vi "RXMux-DM.vi"(0 "Input of RXMux":cluster{"Channe to  Select":u8} {"Channe to  Select" items=["Read Channel", "Select Ch1", "Select Ch2", "Select Ch3", "Select Ch4"]}, 2 "NXT":T1={"Hardware"="NXT", "Flattened String"=""}, 3 "Input Port":u8=1) -> (1 "Output of RXMux":cluster{"Status":bool}, 4 "NXT dup":T1={"Hardware"="NXT", "Flattened String"=""})   [LabVIEW 2011]
uses:
  <vilib>/NXT/Subs/LVHSConnector.ctl
  <vilib>/NXT/Block Support/HWPage.SensorType.ctl
  <vilib>/NXT/Block Support/HWPage.SensorMode.ctl
panel:
  out "Status":bool
  # "mindsensors.com\nCopyright (c) 2009 by mindsensors.com\nEmail: info (<at>) mindsensors (<dot>) com\n\nThis program is free software. You can redistribute it and/or modify\nit under the terms of the GNU General Public License as published by\nthe Free Software Foundation; version 3 of the License.\nRead the license at: http://www.gnu.org/licenses/gpl.txt"
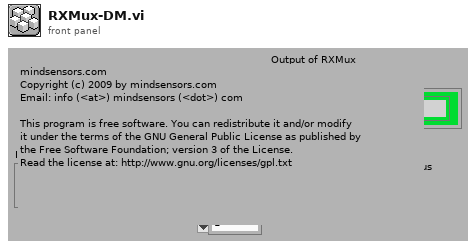
[diagram p1: front panel]
types:
  T1 = typedef "LVHSConnector.ctl" = cluster{"Hardware":string, "Flattened String":string}
  T2 = typedef "HWPage.SensorType.ctl" = u8
  T3 = typedef "HWPage.SensorMode.ctl" = u8
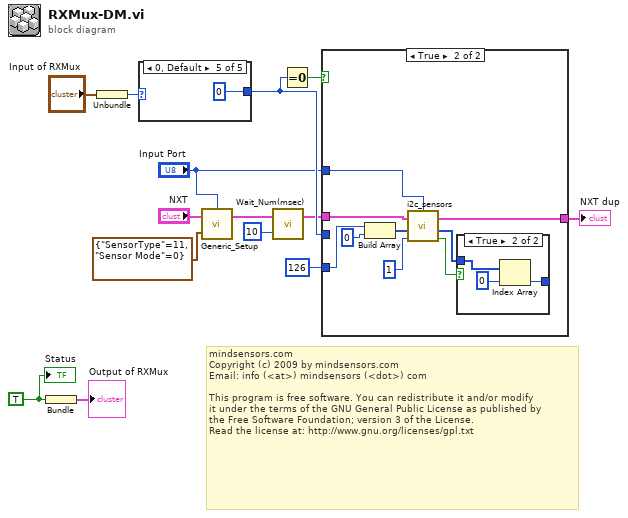
[diagram p0: block diagram]
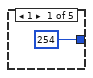
[diagram p2: hidden frame]
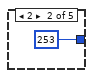
[diagram p3: hidden frame]
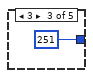
[diagram p4: hidden frame]
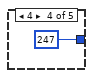
[diagram p5: hidden frame]
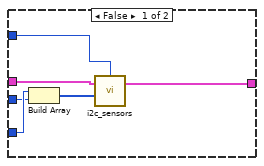
[diagram p6: hidden frame]
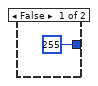
[diagram p7: hidden frame]
diagram:
  w2 = TRUE ("Status")
  # "mindsensors.com\nCopyright (c) 2009 by mindsensors.com\nEmail: info (<at>) mindsensors (<dot>) com\n\nThis program is free software. You can redistribute it and/or modify\nit under the terms of the GNU General Public License as published by\nthe Free Software Foundation; version 3 of the License.\nRead the license at: http://www.gnu.org/licenses/gpl.txt"
  n1 = Bundle("Status"=w2) -> (→"Output of RXMux":cluster{"Status":bool})  [unwired: 1 in]
  n2 = Unbundle("Input of RXMux") -> ("Channe to  Select"=w3:u8)
  n3 = case shown="0, Default" w3 {
    tunnel: [254 253 251 247 0] -> w12
    frame 1 {
    }
    frame 2 {
    }
    frame 3 {
    }
    frame 4 {
    }
    frame 0, Default {
    }
  }
  n4 = call <vilib>:"Generic_Setup.vi"("Sensor Setup"=cluster{"SensorType":T2, "Sensor Mode":T3} {"SensorType"=11, "Sensor Mode"=0}, "NXT"="NXT", "Port"="Input Port") -> ("NXT"=w8:T1)  [unwired: 1 out]
  n5 = call <vilib>:"Wait_Num(msec).vi"("Time (100 msec)"=u8 10 ("Delay"), "NXT"=w8) -> ("NXT"=w6:T1)  [unwired: 2 in]
  n6 = Equal To 0?(x=w12) -> (x = 0?=w13:bool)
  n7 = case shown="True" w13 {
    tunnel: "Input Port" -> [w25 w26]
    tunnel: u8 126 ("Address") -> [w23 w30]
    tunnel: w12 -> [w22 _]
    tunnel: w6 -> [w24 w34]
    tunnel: [w20 w33] -> w5
    frame False {
      n8 = Build Array(w23, w22) -> (w21:i32[])
      n9 = call <vilib>:"i2c_sensors.vi"("Bytes to Write"=w21, "NXT"=w24, "Port"=w25) -> ("NXT"=w20:T1)  [unwired: 2 in, 2 out]
    }
    frame True {
      n10 = Build Array(w30, u8 0 ("register")) -> (w32:u8[])
      n11 = call <vilib>:"i2c_sensors.vi"("Return Length"=u8 1 ("ReturnLength"), "Bytes to Write"=w32, "NXT"=w34, "Port"=w26) -> ("Success?"=w28:bool, "Bytes read"=w27:u8[], "NXT"=w33:T1)  [unwired: 1 in]
      n12 = case shown="True" w28 {
        tunnel: w27 -> [_ w37]
        tunnel: [u8 255 w36] -> _
        frame False {
        }
        frame True {
          n13 = Index Array(array=w37, index=0) -> (element=w36:u8)
        }
      }
    }
  }
  "NXT dup" <- w5
  "Status" <- w2
